vi "Wait for Temperature Setpoint.vi"(6 "Channel":i32, 8 "error in (no error)":errorcluster, 10 "Setpoint (K)":dbl, 11 "Instrument.Cryostat in":refnum<class "Instrument.Cryostat.lvclass">) -> (0 "error out":errorcluster, 3 "Instrument.Cryostat out":refnum<class "Instrument.Cryostat.lvclass">)   [LabVIEW 2016, in "Instrument.Cryostat.lvclass"]
uses:
  Instrument.Cryostat.lvclass
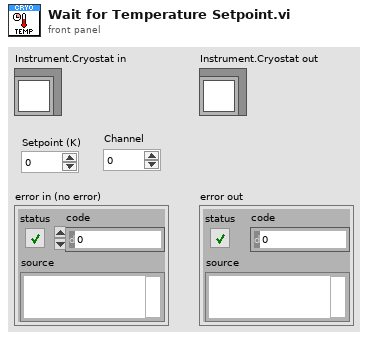
[diagram p1: front panel]
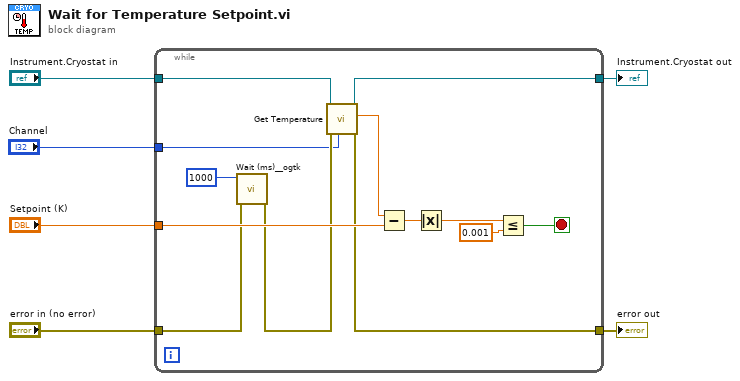
[diagram p0: block diagram]
diagram:
  n1 = while {
    tunnel: "Setpoint (K)" -> [w16]
    tunnel: "Instrument.Cryostat in" -> [w9]
    tunnel: "error in (no error)" -> [w10]
    tunnel: [w13] -> w5
    tunnel: [w8] -> w6
    tunnel: "Channel" -> [w7]
    stop <- w12 stop-if-true
    n2 = call <userlib>:"Wait (ms)__ogtk.vi"("error in (no error)"=w10, "milliseconds to wait"=u32 1000) -> ("error out"=w14:errorcluster)  [unwired: 8 in, 1 out]
    n3 = call-dynamic "Get Temperature.vi"("Channel"=w7, "error in (no error)"=w14, "Instrument.Cryostat in"=w9) -> ("error out"=w13:errorcluster, "Temperature (K)"=w11:dbl, "Instrument.Cryostat out"=w8:refnum<class "Instrument.Cryostat.lvclass">)  [unwired: 4 in, 2 out]
    n4 = Subtract(x=w11, y=w16) -> (x-y=w19:dbl)
    n5 = Absolute Value(x=w19) -> (abs(x)=w18:dbl)
    n6 = Less Or Equal?(x=w18, y=0.001) -> (x <= y?=w12:bool)
  }
  "Instrument.Cryostat out" <- w6
  "error out" <- w5
